vi "CRYGet Sorted String.vi"(11 "Variables In":string[](array[string])) -> (3 "Variables Out":string[](array[string]))   [LabVIEW 2013]
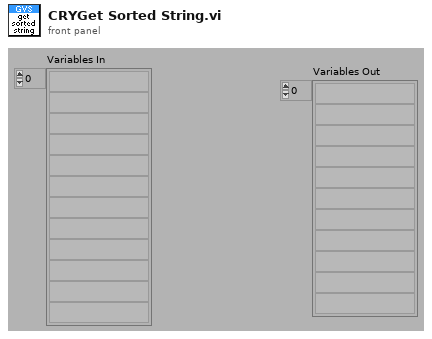
[diagram p1: front panel]
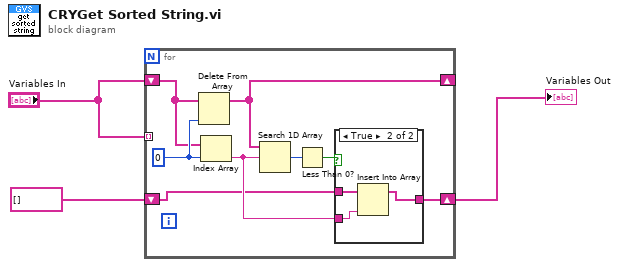
[diagram p0: block diagram]
diagram:
  n1 = for {
    tunnel: "Variables In" -> [_] mode=indexing
    shift-right: [w6] -> _
    shift-left: "Variables In" -> [w8]
    shift-right: [w4] -> w1
    shift-left: string[] [] ("Variables In") -> [w5]
    w9 = 0 ("index")
    n2 = Delete From Array(array=w8, index=w9) -> (array with subset deleted=w6:string[])  [unwired: 1 in, 1 out]
    n3 = Index Array(array=w8, index=w9) -> (element=w7:string)
    n4 = Search 1D Array(1D array=w6, element=w7) -> (index of element=w10:i32)  [unwired: 1 in]
    n5 = Less Than 0?(x=w10) -> (x < 0?=w11:bool)
    n6 = case shown="True" w11 {
      tunnel: w7 -> [_ w15]
      tunnel: w5 -> [w12 w14]
      tunnel: [w12 w13] -> w4
      frame False {
      }
      frame True {
        n7 = Insert Into Array(array=w14, new element=w15) -> (w13:string[])  [unwired: 1 in]
      }
    }
  }
  "Variables Out" <- w1
